vi "From Value.vi"(8 "error in (no error)":errorcluster, 10 "PV Data in":refnum<class "PV Data.lvclass">, 11 "NT Scalar in":refnum<class "NT Scalar.lvclass">) -> (0 "error out":errorcluster, 2 "PV Data out":refnum<class "PV Data.lvclass">, 3 "NT Scalar out":refnum<class "NT Scalar.lvclass">)   [LabVIEW 2020, in "PV Access.lvlib" / "PV Data.lvlib" / "NT Scalar.lvclass"]
uses:
  NT Scalar.lvclass
  NT Scalar.lvclass/NT Scalar.ctl
  PV Data/PV Data.lvclass
  NT Base/NT Base.lvclass
  PV Data/Read Field (Variant).vi
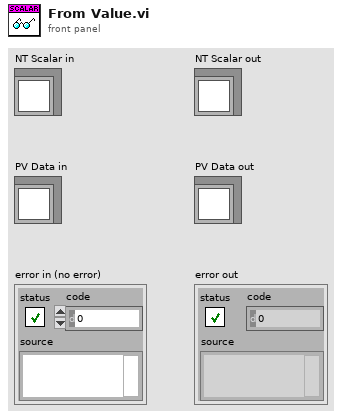
[diagram p1: front panel]
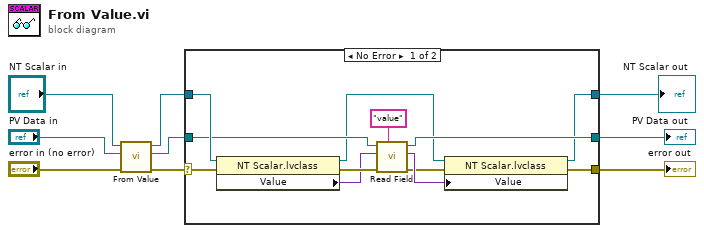
[diagram p0: block diagram]
diagram:
  n1 = call-parent "From Value.vi"("error in (no error)"="error in (no error)", "PV Data in"="PV Data in", "NT Base in"="NT Scalar in") -> ("error out"=w5:errorcluster, "PV Data out"=w1:refnum<class "PV Data.lvclass">, "NT Base out"=w2:refnum<class "NT Scalar.lvclass">)  [unwired: 6 in]
  n2 = case shown="No Error" w5 {
    selector: w5 -> [w21 w22]
    tunnel: [w12 w22] -> w9
    tunnel: [w15 w23] -> w8
    tunnel: [w10 w24] -> w7
    tunnel: w1 -> [w16 w23]
    tunnel: w2 -> [w20 w24]
    frame No Error {
      n3 = property class="NT Scalar.lvclass"(reference=w20, error in=w21) -> (reference out=w11:refnum<class "NT Scalar.lvclass">, error out=w18:errorcluster, "Value"=w17:variant)
      n4 = call-poly "Read Field.vi"("field name"="value", "error in (no error)"=w18, "value"=w17, "PV Data in"=w16) -> ("error out"=w13:errorcluster, "value out"=w14:variant, "PV Data out"=w15:refnum<class "PV Data.lvclass">)  [unwired: 4 in, 1 out]
      n5 = property class="NT Scalar.lvclass"(reference=w11, error in=w13, "Value"=w14) -> (reference out=w10:refnum<class "NT Scalar.lvclass">, error out=w12:errorcluster)
    }
    frame Error {
    }
  }
  "error out" <- w9
  "NT Scalar out" <- w7
  "PV Data out" <- w8
